vi "FRCts20_WebMethods_EscapeHtmlBrackets.vi"(8 "error in (no error)":errorcluster, 10 "HTML String In":string="<!DOCTYPE html>\n<html>\n<head>\n<script>\nfunction open_win() \n{\nwindow.open(\"http://www.w3schools.com\");\n}\n</script>\n</head>\n\n<body>\n<form>\n<input type=\"button\" value=\"Open Window\" onclick=\"open_win()\">\n</form>\n</body>\n\n</html>\n") -> (0 "error out":errorcluster, 2 "result string":string)   [LabVIEW 2013, in "FRCts20_WebMethods.lvlib"]
uses:
  FRCts20_WebMethods.lvlib
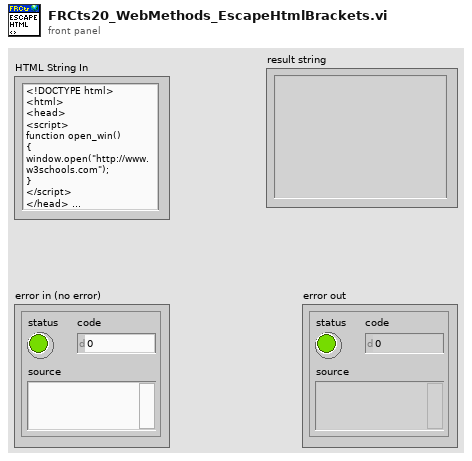
[diagram p1: front panel]
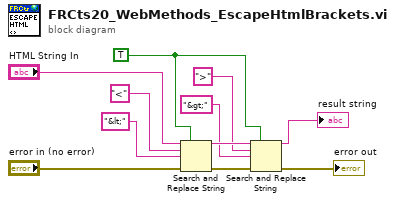
[diagram p0: block diagram]
diagram:
  w8 = TRUE ("replace all? (F)")
  n1 = Search and Replace String(replace all?=w8, input string="HTML String In", search string="<", replace string="&lt;" ("replace string (\"\")"), error in="error in (no error)") -> (result string=w9:string, error out=w7:errorcluster)  [unwired: 3 in, 2 out]
  n2 = Search and Replace String(replace all?=w8, input string=w9, search string=">", replace string="&gt;" ("replace string (\"\")"), error in=w7) -> (result string=→"result string":string, error out=→"error out":errorcluster)  [unwired: 3 in, 2 out]
